vi "Extend Chunk into Schedule.vi"(11 "Array in":u32[](array[numeric])) -> (3 "Array out":u32[](array[numeric]) format="%08x")   [LabVIEW 2012, in "SHA256.lvlib"]
doc: "In the SHA-256 algorithm, each block of 16 words (512 bits) is first extened into a schedule of 64 32bit words, mixing up the bits of the 16 words of the block into the extra words."
uses:
  SHA256.lvlib
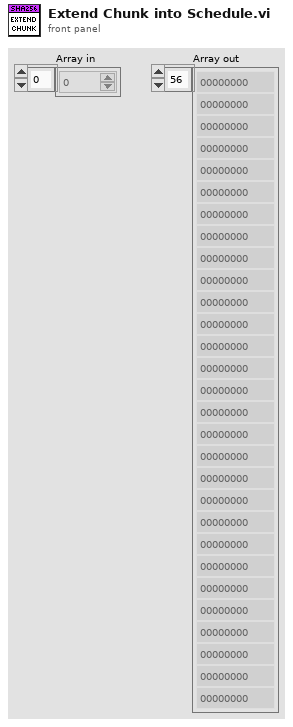
[diagram p1: front panel]
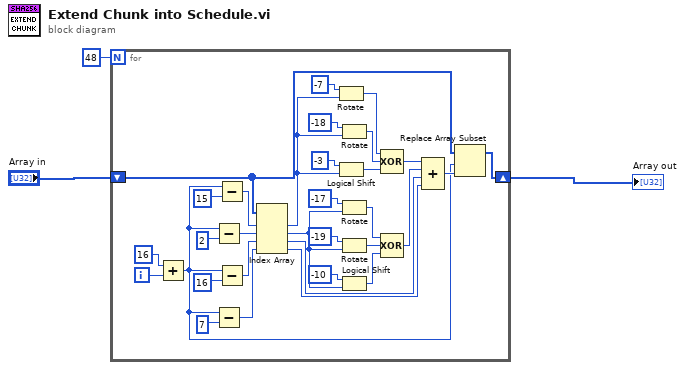
[diagram p0: block diagram]
diagram:
  n1 = for {
    N: 48 -> [_]
    shift-right: [w6] -> w3
    shift-left: "Array in" -> [w29]
    i -> [w35]
    n2 = Add(x=16, y=w35) -> (x+y=w4:i32)
    n3 = Subtract(x=w4, y=2) -> (x-y=w31:i32)
    n4 = Subtract(x=w4, y=7) -> (x-y=w25:i32)
    n5 = Subtract(x=w4, y=15) -> (x-y=w33:i32)
    n6 = Subtract(x=w4, y=16) -> (x-y=w28:i32)
    n7 = Index Array(array=w29, index #1=w33, index #2=w31, index #3=w28, index #4=w25) -> (element #1=w22:u32, element #2=w15:u32, element #3=w8:u32, element #4=w7:u32)
    n8 = Rotate(1:w22, 2:i16 -7 ("y")) -> (0:w20:u32)
    n9 = Logical Shift(y=i16 -3, x=w22) -> (x << y=w18:u32)
    n10 = Rotate(1:w22, 2:i16 -18 ("y")) -> (0:w19:u32)
    n11 = Rotate(1:w15, 2:i16 -17 ("y")) -> (0:w11:u32)
    n12 = Rotate(1:w15, 2:i16 -19 ("y")) -> (0:w12:u32)
    n13 = Logical Shift(y=i16 -10, x=w15) -> (x << y=w13:u32)
    n14 = Compound Arithmetic op=XOR(w20, w19, w18) -> (w10:u32)
    n15 = Compound Arithmetic op=XOR(w11, w12, w13) -> (w9:u32)
    n16 = Compound Arithmetic op=ADD(w10, w9, w8, w7) -> (w5:u32)
    n17 = Replace Array Subset(array=w29, new element=w5, index=w4) -> (w6:u32[])
  }
  "Array out" <- w3
